vi "DSOX2014A setup subVI.vi"(8 "error in (no error)":errorcluster, 11 "VISA Refnum in":refnum<visa-resource-name>) -> (0 "error out":errorcluster, 3 "VISA Refnum out":refnum<visa-resource-name>)   [LabVIEW 2016]
uses:
  <instrlib>/Agilent 2000 3000 X-Series/Public/Configure/Configure Timebase (Basic).vi
  <instrlib>/Agilent 2000 3000 X-Series/Agilent 2000 3000 X-Series.lvlib
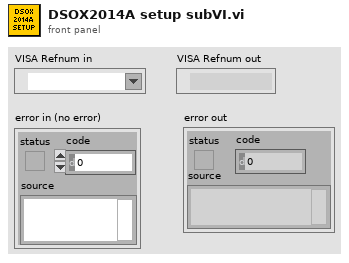
[diagram p1: front panel]
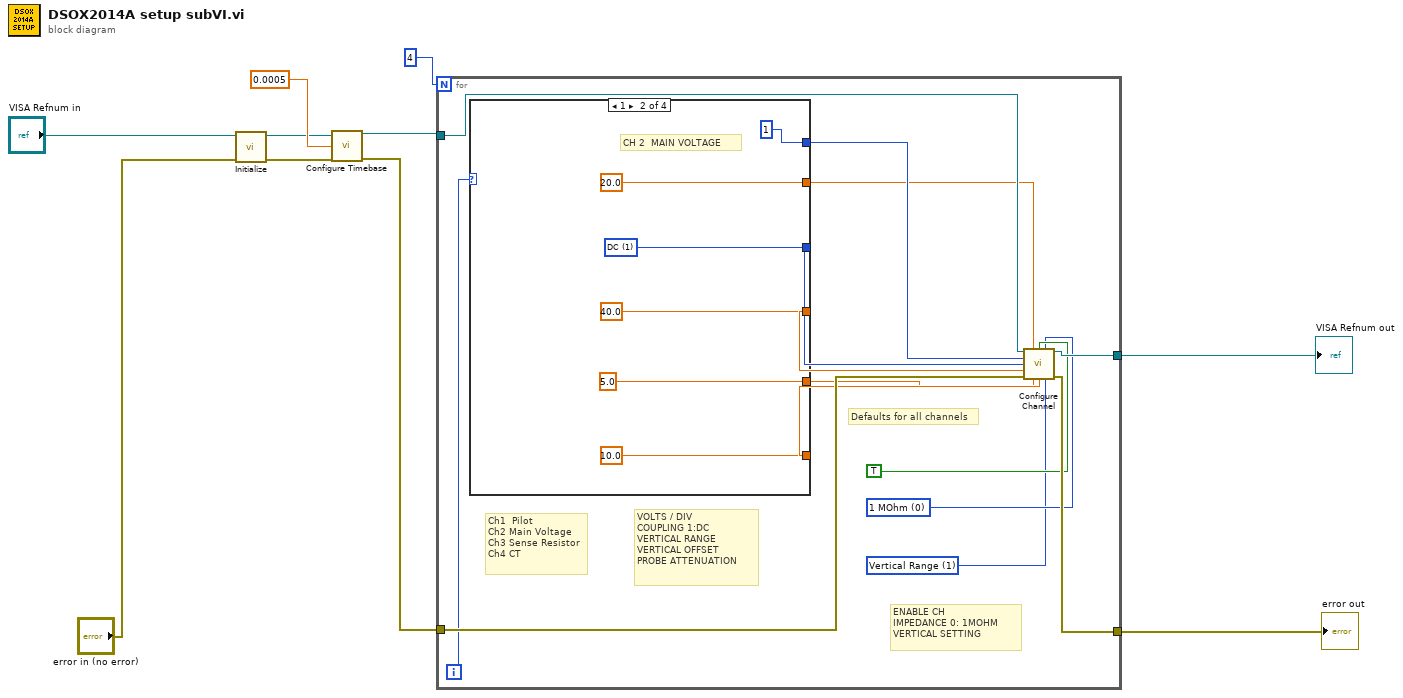
[diagram p0: block diagram]
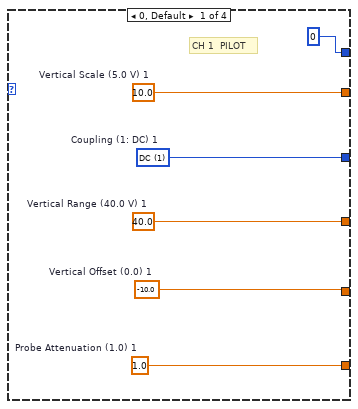
[diagram p2: hidden frame]
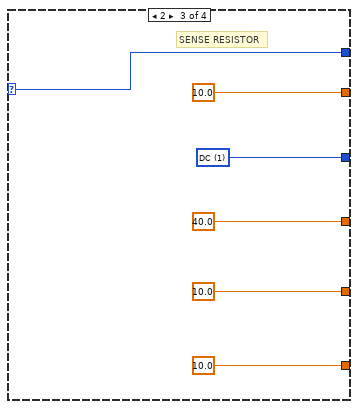
[diagram p3: hidden frame]
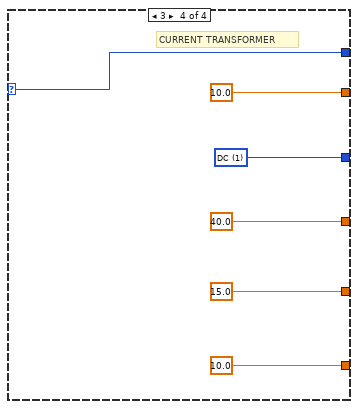
[diagram p4: hidden frame]
diagram:
  n1 = call <instrlib>:"Initialize.vi"("error in (no error)"="error in (no error)", "VISA resource name"="VISA Refnum in") -> ("error out"=w2:errorcluster, "VISA resource name out"=w4:refnum<visa-resource-name>)  [unwired: 8 in]
  n2 = call-poly <instrlib>:"Configure Timebase.vi"("VISA resource name"=w4, "Scale (50 s/div)"=0.0005, "error in (no error)"=w2) -> ("VISA resource name out"=w3:refnum<visa-resource-name>, "error out"=w1:errorcluster)  [unwired: 11 in]
  n3 = for {
    N: 4 -> [_]
    tunnel: w3 -> [w20]
    tunnel: w1 -> [w24]
    tunnel: [w23] -> w8
    tunnel: [w22] -> w10
    i -> [w16]
    w17 = 1 items=["Vertical Scale", "Vertical Range"] ("Vertical Setting (1: Vertical Range)")
    w18 = 0 items=["1 MOhm", "50 Ohm"] ("Impedance (0: 1 MOhm)")
    # "ENABLE CH\nIMPEDANCE 0: 1MOHM\nVERTICAL SETTING"
    # "VOLTS / DIV\nCOUPLING 1:DC\nVERTICAL RANGE\nVERTICAL OFFSET\nPROBE ATTENUATION"
    # "Defaults for all channels"
    # "Ch1  Pilot\nCh2 Main Voltage\nCh3 Sense Resistor\nCh4 CT"
    n4 = case shown="1" w16 {
      selector: w16 -> [_ _ w37 w43]
      tunnel: [0 1 w37 w43] -> w21
      tunnel: [w29 20.0 ("Vertical Scale (5.0 V) 2") 10.0 ("Vertical Scale (5.0 V) 3") 10.0 ("Vertical Scale (5.0 V) 4")] -> w11
      tunnel: [w28 w34 w41 w47] -> w12
      tunnel: [w27 40.0 ("Vertical Range (40.0 V) 2") 40.0 ("Vertical Range (40.0 V) 3") 40.0 ("Vertical Range (40.0 V) 4")] -> w13
      tunnel: [w26 5.0 ("Vertical Offset (0.0) 2") 10.0 ("Vertical Offset (0.0) 3") 15.0 ("Vertical Offset (0.0) 4")] -> w14
      tunnel: [w25 10.0 ("Probe Attenuation (1.0) 2") 10.0 ("Probe Attenuation (1.0) 3") 10.0 ("Probe Attenuation (1.0) 4")] -> w15
      frame 0, Default {
        w27 = 40.0  # Vertical Range (40.0 V) 1
        w28 = 1 items=["AC", "DC"]  # Coupling (1: DC) 1
        w29 = 10.0  # Vertical Scale (5.0 V) 1
        w25 = 1.0  # Probe Attenuation (1.0) 1
        w26 = -10.0  # Vertical Offset (0.0) 1
        # "CH 1  PILOT"
      }
      frame 1 {
        w34 = 1 items=["AC", "DC"] ("Coupling (1: DC) 2")
        # "CH 2  MAIN VOLTAGE"
      }
      frame 2 {
        w41 = 1 items=["AC", "DC"] ("Coupling (1: DC) 3")
        # "SENSE RESISTOR"
      }
      frame 3 {
        w47 = 1 items=["AC", "DC"] ("Coupling (1: DC) 4")
        # "CURRENT TRANSFORMER"
      }
    }
    n5 = call <instrlib>:"Configure Channel.vi"("VISA resource name"=w20, "Vertical Scale (5.0 V)"=w11, "Enable Channel (T: Enable)"=TRUE, "Impedance (0: 1 MOhm)"=w18, "Channel Name (0: Channel 1)"=w21, "Coupling (1: DC)"=w12, "Vertical Range (40.0 V)"=w13, "error in (no error)"=w24, "Vertical Offset (0.0)"=w14, "Probe Attenuation (1.0)"=w15, "Vertical Setting (1: Vertical Range)"=w17) -> ("VISA resource name out"=w22:refnum<visa-resource-name>, "error out"=w23:errorcluster)  [unwired: 3 in]
  }
  "error out" <- w8
  "VISA Refnum out" <- w10
